vi "Main.vi"(8 "error in (no error)":errorcluster, 11 "Piezo in":refnum<class "Piezo.lvclass">) -> (0 "error out":errorcluster, 3 "component":refnum<class "Piezo.lvclass">)   [LabVIEW 2012, in "Piezo.lvclass"]
doc: "Main VI of the component. This should contain the GUI of your component and be called when creating an executable."
uses:
  Piezo.lvclass
  <vilib>/Distrio/Murmex/Murmex/command_enum.ctl
  <vilib>/Distrio/Murmex/InitialiseMessage/InitialiseMessage.lvclass
  <vilib>/Distrio/Murmex/GenericMessage/GenericMessage.lvclass
  <vilib>/Distrio/Murmex/TerminateMessage/TerminateMessage.lvclass
  <vilib>/Distrio/Murmex/ConfigureMessage/ConfigureMessage.lvclass
  <vilib>/Distrio/Murmex/Murmex/update_cluster.ctl
  Piezo.lvclass/Piezo.ctl
  <vilib>/Distrio/Murmex/Murmex/Murmex.lvclass
  <vilib>/Distrio/Murmex/Murmex/Set configure at initialise.vi
  <vilib>/Distrio/Murmex/Murmex/Set log reference.vi
  <vilib>/Distrio/Murmex/Murmex/Set VI reference.vi
  <vilib>/Distrio/Murmex/Murmex/Get ID.vi
  <vilib>/Distrio/Murmex/Murmex/Set write log to disk.vi
  <vilib>/Distrio/Murmex/Message/Message.lvclass
panel:
  out "Piezo position chart":dbl[unit](graph)
  in  "button:configure":bool
  in  "Tab Control":enum32{"User", "Debug"}(tab)
  in  "position log?":bool
  in  "button:forward":bool
  in  "button:backward":bool
  out "Output voltage":dbl[unit]
  in  "Step size":dbl[unit]
  in  "Piezo position":dbl[unit]
  in  "button:send command":bool
  in  "command":T1
  in  "generic command":string
  in  "button:quit":bool
  in  "terminate?":bool
  out "log":string
  in  "Component id":string="Piezo"
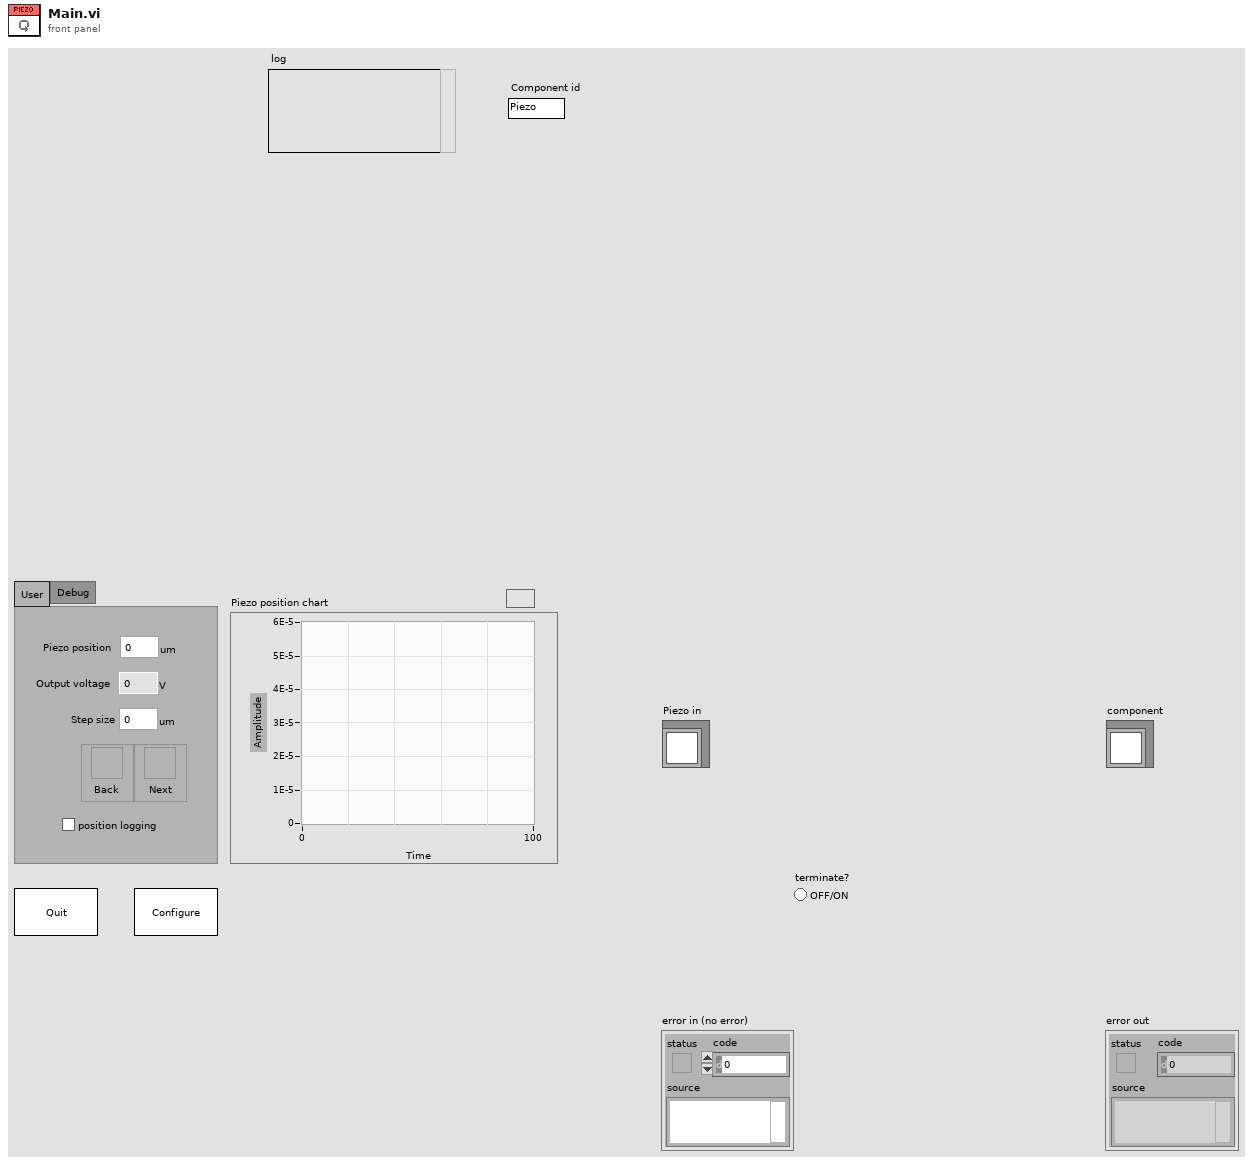
[diagram p1: front panel]
types:
  T1 = typedef "Murmex.lvlib/Murmex.lvclass/command_enum.ctl" = enum16{"null", "initialise", "reset", "terminate", "acknowledge", "update", "inspect", "inform", "proceed", "start", "stop", "fetch", "configure", "generic"}
  T2 = enum8{"Enabled", "Disabled", "Disabled and Grayed Out"}
  T3 = typedef "Murmex.lvlib/Murmex.lvclass/update_cluster.ctl" = cluster{"target ID":string, "key chains":string[], "values":variant[]}
  T4 = typedef "Murmex.lvclass/command_enum.ctl" = enum16{"null", "initialise", "reset", "terminate", "acknowledge", "update", "inspect", "inform", "proceed", "start", "stop", "fetch", "configure", "generic"}
  T5 = typedef "Murmex.lvclass/Event type enumerations.ctl" = enum16{"before", "after"}
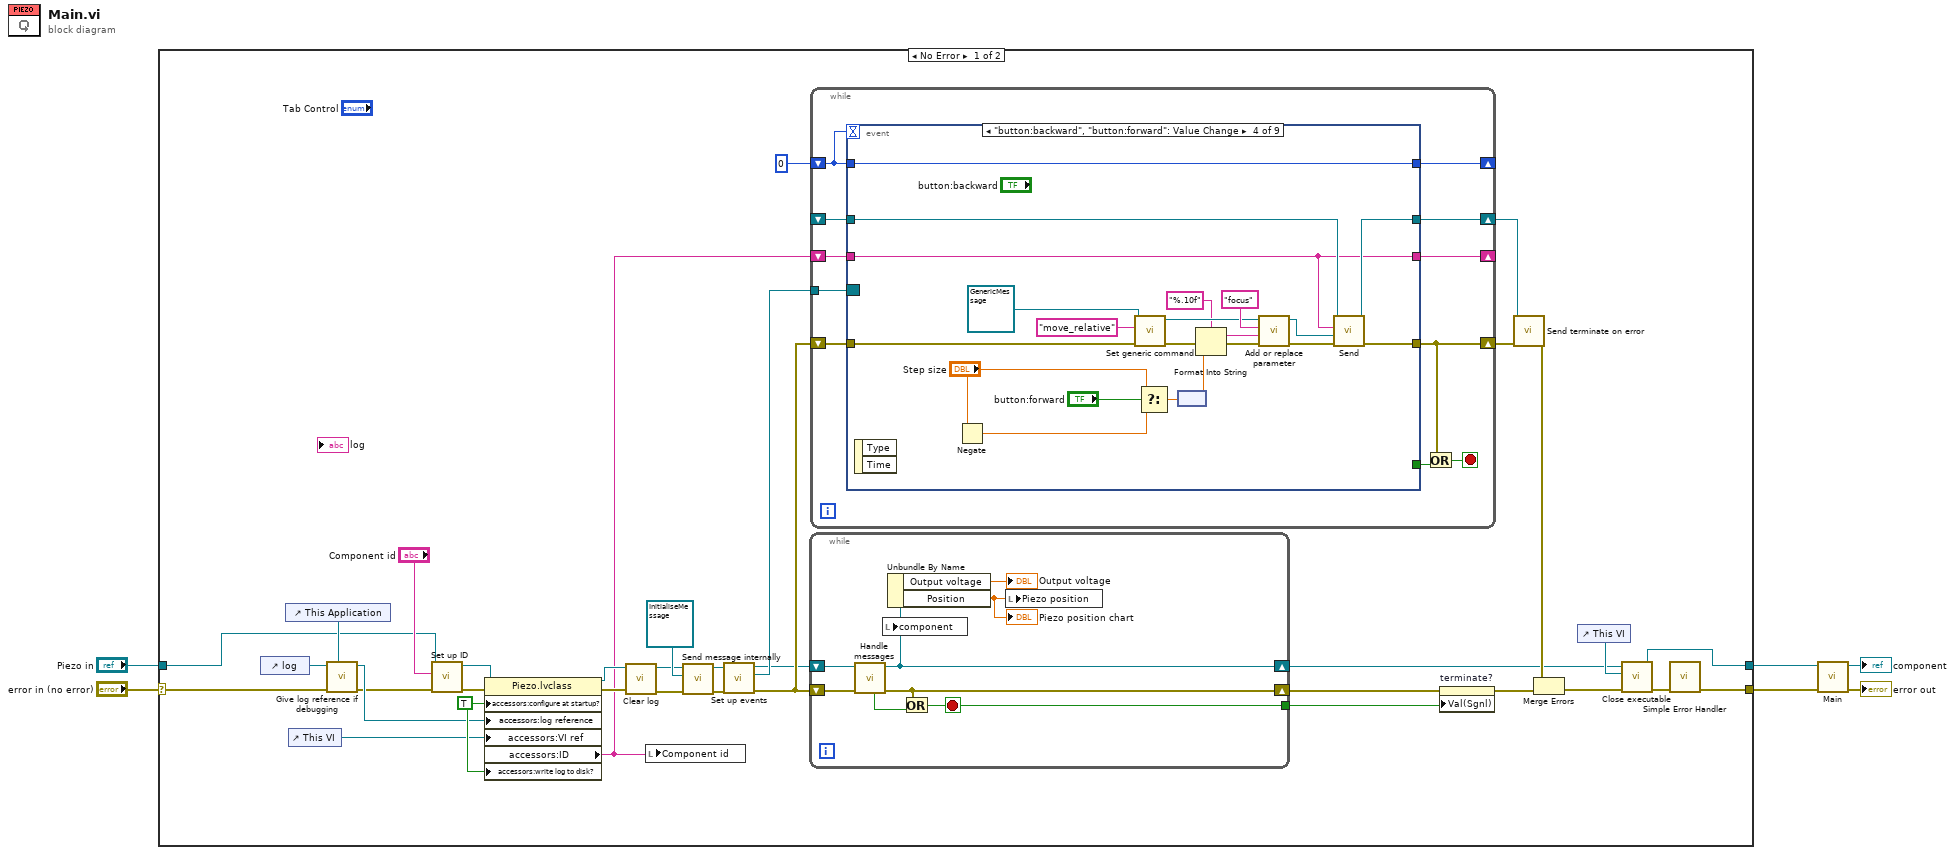
[diagram p0: block diagram]
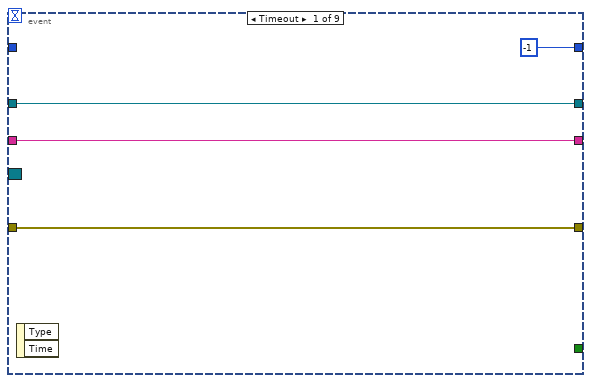
[diagram p2: hidden frame]
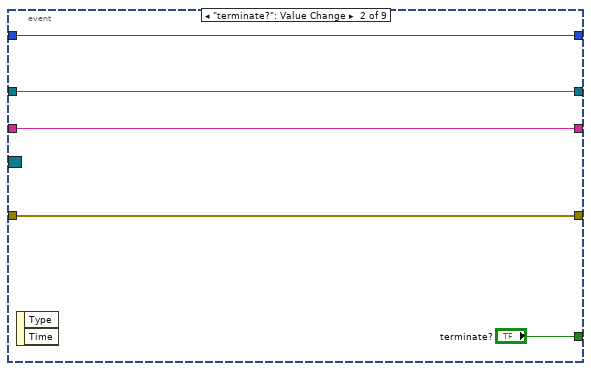
[diagram p3: hidden frame]
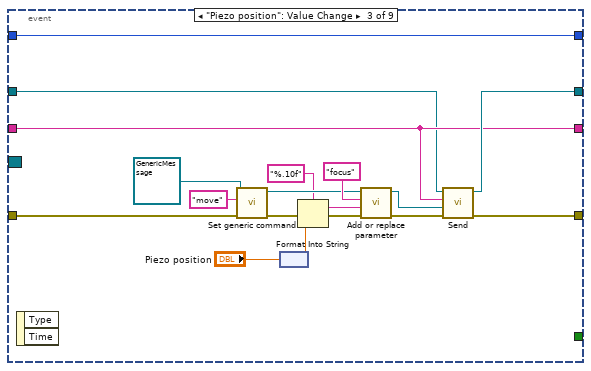
[diagram p4: hidden frame]
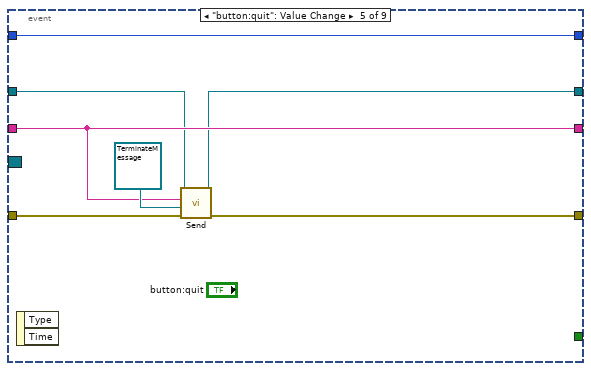
[diagram p5: hidden frame]
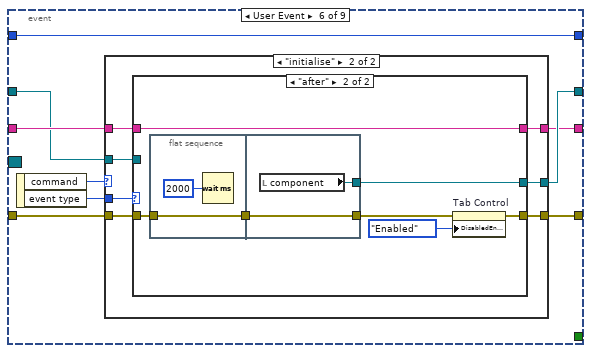
[diagram p6: hidden frame]
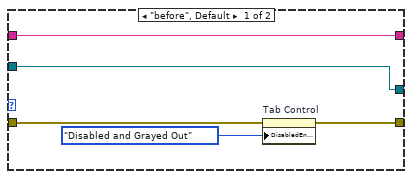
[diagram p8: hidden frame]
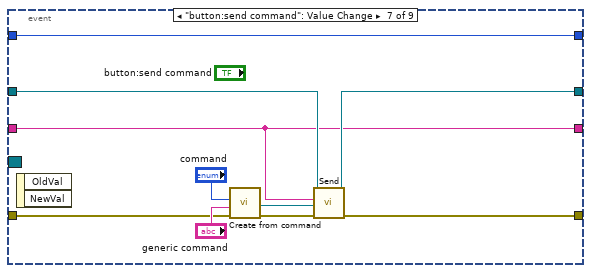
[diagram p9: hidden frame]
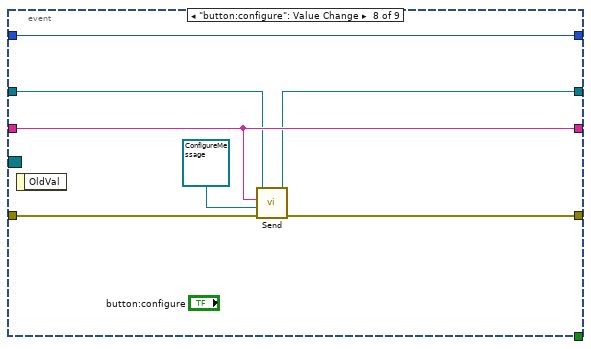
[diagram p10: hidden frame]
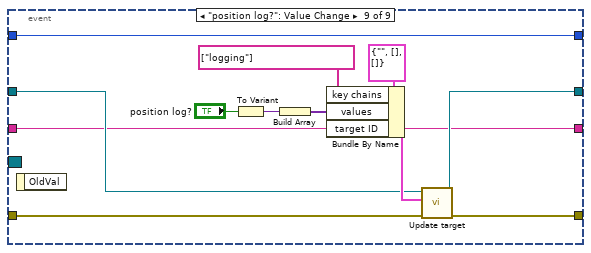
[diagram p11: hidden frame]
diagram:
  n1 = case shown="No Error" "error in (no error)" {
    selector: "error in (no error)" -> [w25 w181]
    tunnel: [w10 w181] -> w3
    tunnel: [w8 w180] -> w2
    tunnel: "Piezo in" -> [w24 w180]
    frame No Error {
      w41 = TRUE ("configure at startup?")
      n2 = control-ref of="log"() -> (w32:refnum<vi>)
      n3 = control-ref of="This Application"() -> (w26:refnum<vi>)
      n4 = control-ref of="This VI"() -> (w33:refnum<vi>)
      n5 = call "Give log reference if debugging.vi"("application ref"=w26, "error in (no error)"=w25, "log reference in"=w32) -> ("error out"=w27:errorcluster, "log reference out"=w31:refnum<vi>)  [unwired: 6 in, 1 out]
      n6 = call <vilib>:"Set up ID.vi"("error in (no error)"=w27, "component ID"="Component id", "MurmexBase in"=w24) -> ("error out"=w29:errorcluster, "MurmexBase out"=w30:refnum<class "Piezo.lvclass">)  [unwired: 6 in, 1 out]
      n7 = property class="Piezo.lvclass"(reference=w30, error in=w29, "accessors:configure at startup?"=w41, "accessors:log reference"=w31, "accessors:VI ref"=w33, "accessors:write log to disk?"=w41) -> (reference out=w40:refnum<class "Piezo.lvclass">, error out=w38:errorcluster, "accessors:ID"=w22:string)
      n8 = call <vilib>:"Clear log.vi"("error in (no error)"=w38, "MurmexBase in"=w40) -> ("error out"=w35:errorcluster, "MurmexBase out"=w34:refnum<class "Piezo.lvclass">)  [unwired: 8 in]
      n9 = local write "Component id"(w22) -> ()
      n10 = call <vilib>:"Send message internally.vi"("error in (no error)"=w35, "Message"=refnum<class "InitialiseMessage.lvclass"> refnum ("InitialiseMessage"), "Murmex in"=w34) -> ("error out"=w36:errorcluster, "Murmex out"=w37:refnum<class "Piezo.lvclass">)  [unwired: 7 in]
      n11 = call <vilib>:"Set up events.vi"("error in (no error)"=w36, "MurmexBase in"=w37) -> ("error out"=w23:errorcluster, "Event Registration Refnum"=w20:refnum<event-registration>, "MurmexBase out"=w7:refnum<class "Piezo.lvclass">)  [unwired: 7 in]
      n12 = while {
        shift-right: [w174] -> w9
        shift-left: w7 -> [w179]
        shift-right: [w176] -> w19
        shift-left: w23 -> [w178]
        tunnel: [w175] -> w18
        stop <- w175 stop-if-true
        n13 = call <vilib>:"Handle messages.vi"("error in (no error)"=w178, "Murmex in"=w179) -> ("error out"=w176:errorcluster, "Murmex out"=w174:refnum<class "Piezo.lvclass">, "terminated?"=w177:bool)  [unwired: 7 in]
        n14 = local write "component"(w174) -> ()
        n15 = Unbundle By Name(w174) -> ("Output voltage"=→"Output voltage":dbl[unit], "Position"=w172:dbl[unit])
        "Piezo position chart" <- w172
        n16 = Or(x=w176, y=w177) -> (x .or. y?=w175:bool)
        n17 = local write "Piezo position"(w172) -> ()
      }
      n18 = while {
        shift-right: [w46] -> w11
        shift-left: w23 -> [w50]
        shift-right: [w49] -> _
        shift-left: w22 -> [w48]
        shift-right: [w51] -> _
        shift-left: 0 -> [w52]
        tunnel: w20 -> [w44]
        shift-right: [w43] -> w12
        shift-left: _ -> [w42]
        stop <- w47 stop-if-true
        n19 = event shown="[3] \"button:backward\", \"button:forward\": Value Change" {
          selector: w44 -> [_ _ _ _ _ _ _ _ _]
          dyn-events: _ -> [_ _ _ _ _ _ _ _ _]
          timeout: w52 -> [_ _ _ _ _ _ _ _ _]
          tunnel: w52 -> [_ w58 w79 w88 w105 w108 w143 w155 w171]
          tunnel: [-1 w58 w79 w88 w105 w108 w143 w155 w171] -> w51
          tunnel: [w56 w60 w78 w89 w106 w113 w147 w158 w161] -> w46
          tunnel: w50 -> [w56 w60 w76 w90 w107 w114 w148 w159 w162]
          tunnel: [w54 w59 w66 w85 w103 w111 w144 w156 w160] -> w49
          tunnel: w48 -> [w54 w59 w66 w85 w103 w110 w144 w156 w160]
          tunnel: [_ "terminate?" _ _ _ _ _ _ _] -> w45
          tunnel: [w55 w57 w77 w86 w101 w112 w145 w153 w163] -> w43
          tunnel: w42 -> [w55 w57 w65 w87 w102 w109 w146 w154 w164]
          event Timeout {
            n20 = event-data() -> ()  [unwired: 1 in, 2 out]
          }
          event "terminate?": Value Change {
            n21 = event-data() -> ()  [unwired: 1 in, 2 out]
          }
          event "Piezo position": Value Change {
            n22 = event-data() -> ()  [unwired: 1 in, 2 out]
            n23 = call <vilib>:"Set generic command.vi"("error in (no error)"=w76, "generic command"="move", "GenericMessage in"=refnum<class "GenericMessage.lvclass"> refnum ("Message in")) -> ("error out"=w70:errorcluster, "GenericMessage out"=w68:refnum<class "GenericMessage.lvclass">)  [unwired: 7 in]
            n24 = node("Piezo position") -> (w63:dbl)
            n25 = Format Into String(format string="%.10f", error in=w70, w63) -> (resulting string=w72:string, error out=w71:errorcluster)  [unwired: 1 in]
            n26 = call <vilib>:"Add or replace parameter.vi"("error in (no error)"=w71, "value"=w72, "name"="focus", "Message in"=w68) -> ("error out"=w69:errorcluster, "Message out"=w67:refnum<class "GenericMessage.lvclass">)  [unwired: 6 in]
            n27 = call <vilib>:"Send.vi"("error in (no error)"=w69, "Message"=w67, "recipient"=w66, "Murmex in"=w65) -> ("error out"=w78:errorcluster, "Murmex out"=w77:refnum<class "Murmex.lvclass">)  [unwired: 6 in]
          }
          event "button:backward", "button:forward": Value Change {
            n28 = event-data() -> ()  [unwired: 1 in, 2 out]
            n29 = Negate(x="Step size") -> (-x=w82:dbl[unit])
            n30 = call <vilib>:"Set generic command.vi"("error in (no error)"=w90, "generic command"="move_relative", "GenericMessage in"=refnum<class "GenericMessage.lvclass"> refnum ("Message in")) -> ("error out"=w95:errorcluster, "GenericMessage out"=w93:refnum<class "GenericMessage.lvclass">)  [unwired: 7 in]
            n31 = Select(t="Step size", s="button:forward", f=w82) -> (s? t:f=w81:dbl[unit])
            n32 = node(w81) -> (w91:dbl)
            n33 = Format Into String(format string="%.10f", error in=w95, w91) -> (resulting string=w97:string, error out=w96:errorcluster)  [unwired: 1 in]
            n34 = call <vilib>:"Add or replace parameter.vi"("error in (no error)"=w96, "value"=w97, "name"="focus", "Message in"=w93) -> ("error out"=w94:errorcluster, "Message out"=w92:refnum<class "GenericMessage.lvclass">)  [unwired: 6 in]
            n35 = call <vilib>:"Send.vi"("error in (no error)"=w94, "Message"=w92, "recipient"=w85, "Murmex in"=w87) -> ("error out"=w89:errorcluster, "Murmex out"=w86:refnum<class "Murmex.lvclass">)  [unwired: 6 in]
          }
          event "button:quit": Value Change {
            n36 = event-data() -> ()  [unwired: 1 in, 2 out]
            n37 = call <vilib>:"Send.vi"("error in (no error)"=w107, "Message"=refnum<class "TerminateMessage.lvclass"> refnum ("TerminateMessage"), "recipient"=w103, "Murmex in"=w102) -> ("error out"=w106:errorcluster, "Murmex out"=w101:refnum<class "Murmex.lvclass">)  [unwired: 6 in]
          }
          event User Event {
            n38 = event-data() -> ("command"=w116:T4, "event type"=w115:T5)  [unwired: 1 in]
            n39 = case shown="\"initialise\"" w116 {
              tunnel: w115 -> [_ w126]
              tunnel: w114 -> [w117 w125]
              tunnel: [w117 w124] -> w113
              tunnel: [w118 w123] -> w112
              tunnel: [w119 w122] -> w111
              tunnel: w110 -> [w119 w121]
              tunnel: w109 -> [w118 w120]
              frame "null", Default {
              }
              frame "initialise" {
                n40 = case shown="\"after\"" w126 {
                  tunnel: w125 -> [w131 w137]
                  tunnel: [w130 w135] -> w124
                  tunnel: [w128 w133] -> w123
                  tunnel: [w127 w132] -> w122
                  tunnel: w121 -> [w127 w132]
                  tunnel: w120 -> [w128 _]
                  frame "before", Default {
                    n41 = property on="Tab Control" class="TabCtl (strict)"(error in=w131, "DisabledEnum"=T2."Disabled and Grayed Out" ("Disabled")) -> (error out=w130:errorcluster)  [unwired: 1 in, 1 out]
                  }
                  frame "after" {
                    n42 = flat-sequence {
                      tunnel: [w139] -> w138
                      tunnel: w137 -> [w139]
                      tunnel: w138 -> [w142]
                      tunnel: [w142] -> w136
                      tunnel: [w141] -> w133
                      frame #0 {
                        n43 = Wait (ms)(milliseconds to wait=u32 2000) -> ()  [unwired: 1 out]
                      }
                      frame #1 {
                        n44 = local read "component"() -> (w141:refnum<class "Piezo.lvclass">)
                      }
                    }
                    n45 = property on="Tab Control" class="TabCtl (strict)"(error in=w136, "DisabledEnum"=T2."Enabled" ("Disabled")) -> (error out=w135:errorcluster)  [unwired: 1 in, 1 out]
                  }
                }
              }
            }
          }
          event "button:send command": Value Change {
            n46 = event-data() -> ()  [unwired: 1 in, 2 out]
            n47 = call <vilib>:"Create from command.vi"("error in (no error)"=w148, "generic command"="generic command", "command"="command") -> ("error out"=w152:errorcluster, "Message out"=w149:refnum<class "Message.lvclass">)  [unwired: 7 in]
            n48 = call <vilib>:"Send.vi"("error in (no error)"=w152, "Message"=w149, "recipient"=w144, "Murmex in"=w146) -> ("error out"=w147:errorcluster, "Murmex out"=w145:refnum<class "Murmex.lvclass">)  [unwired: 6 in]
          }
          event "button:configure": Value Change {
            n49 = event-data() -> ()  [unwired: 1 in, 1 out]
            n50 = call <vilib>:"Send.vi"("error in (no error)"=w159, "Message"=refnum<class "ConfigureMessage.lvclass"> refnum ("ConfigureMessage"), "recipient"=w156, "Murmex in"=w154) -> ("error out"=w158:errorcluster, "Murmex out"=w153:refnum<class "Murmex.lvclass">)  [unwired: 6 in]
          }
          event "position log?": Value Change {
            n51 = event-data() -> ()  [unwired: 1 in, 1 out]
            n52 = To Variant(anything="position log?") -> (Variant=w166:variant)
            n53 = Build Array(w166) -> (w170:variant[])
            n54 = Bundle By Name(cluster=T3 {"target ID"="", "key chains"=[], "values"=[]} ("update cluster"), "key chains"=string[] ["logging"], "values"=w170, "target ID"=w160) -> (w168:T3)
            n55 = call <vilib>:"Update target.vi"("error in (no error)"=w162, "update cluster"=w168, "MurmexBase in"=w164) -> ("error out"=w161:errorcluster, "MurmexBase out"=w163:refnum<class "Murmex.lvclass">)  [unwired: 7 in]
          }
        }
        n56 = Or(x=w46, y=w45) -> (x .or. y?=w47:bool)
      }
      n57 = property on="terminate?" class="Bool (strict)"(error in=w19, "Val(Sgnl)"=w18) -> (error out=w13:errorcluster)  [unwired: 1 in, 1 out]
      n58 = call <vilib>:"Send terminate on error.vi"("error in (no error)"=w11, "Murmex in"=w12) -> ("error out"=w14:errorcluster)  [unwired: 8 in, 1 out]
      n59 = Merge Errors(w14, w13) -> (w16:errorcluster)
      n60 = control-ref of="This VI"() -> (w15:refnum<vi>)
      n61 = call <vilib>:"Close executable.vi"("error in (no error)"=w16, "main VI ref (optional)"=w15, "MurmexBase in"=w9) -> ("error out"=w17:errorcluster, "MurmexBase out"=w8:refnum<class "Piezo.lvclass">)  [unwired: 7 in]
      n62 = call <vilib>:"Simple Error Handler.vi"("error in (no error)"=w17) -> ("error out"=w10:errorcluster)  [unwired: 4 in, 4 out]
    }
    frame Error {
    }
  }
  n63 = call-parent "Main.vi"("error in (no error)"=w3, "Murmex in"=w2) -> ("error out"=→"error out":errorcluster, "Murmex out"=→"component":refnum<class "Piezo.lvclass">)  [unwired: 8 in]
